vi "446x_AO_MinMax.vi"(2 "AO.Range":T1) -> (6 "AO.min":dbl, 7 "AO.max":dbl)   [LabVIEW 2016]
uses:
  Typedefs/446xAO-enum.ctl
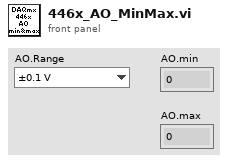
[diagram p1: front panel]
types:
  T1 = typedef "446xAO-enum.ctl" = enum16{"±0.1 V", "±1.0 V", "±10.0 V"}
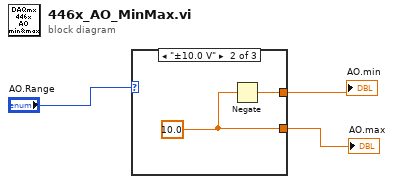
[diagram p0: block diagram]
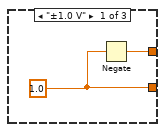
[diagram p2: hidden frame]
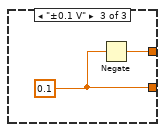
[diagram p3: hidden frame]
diagram:
  n1 = case shown="\"±10.0 V\"" "AO.Range" {
    tunnel: [w5 w7 w9] -> w1
    tunnel: [w4 w6 w8] -> w3
    frame "±1.0 V" {
      w5 = 1.0
      n2 = Negate(x=w5) -> (-x=w4:dbl)
    }
    frame "±10.0 V" {
      w7 = 10.0
      n3 = Negate(x=w7) -> (-x=w6:dbl)
    }
    frame "±0.1 V" {
      w9 = 0.1
      n4 = Negate(x=w9) -> (-x=w8:dbl)
    }
  }
  "AO.min" <- w3
  "AO.max" <- w1
